vi "outPutOneTestCaseInCanFile.vi"(8 "error in":errorcluster, 10 "*varNoRepeatArr":string[](array[string]), 11 "secName":string) -> (0 "error out":errorcluster, 3 "oneTestCaseInCanFile":string[](array[string]))   [LabVIEW 2010]
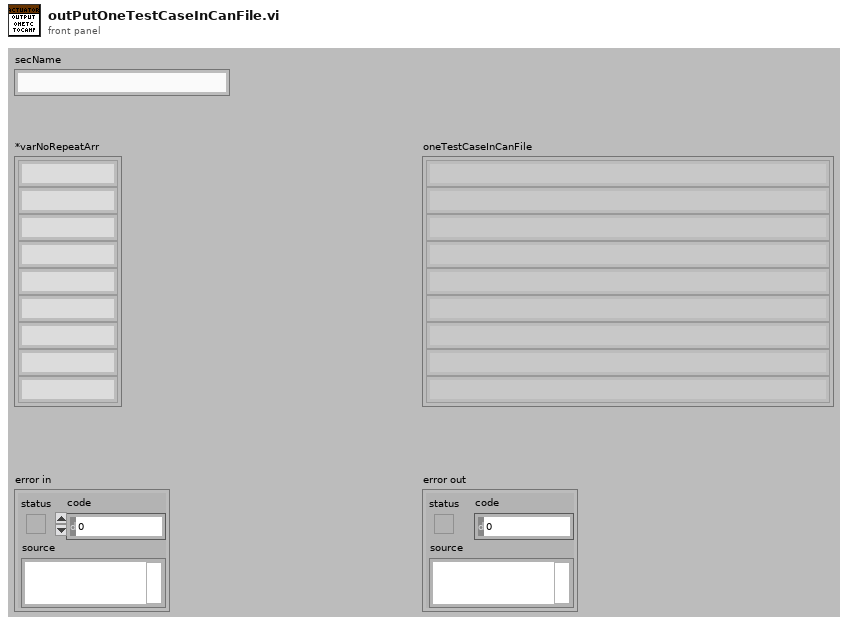
[diagram p1: front panel]
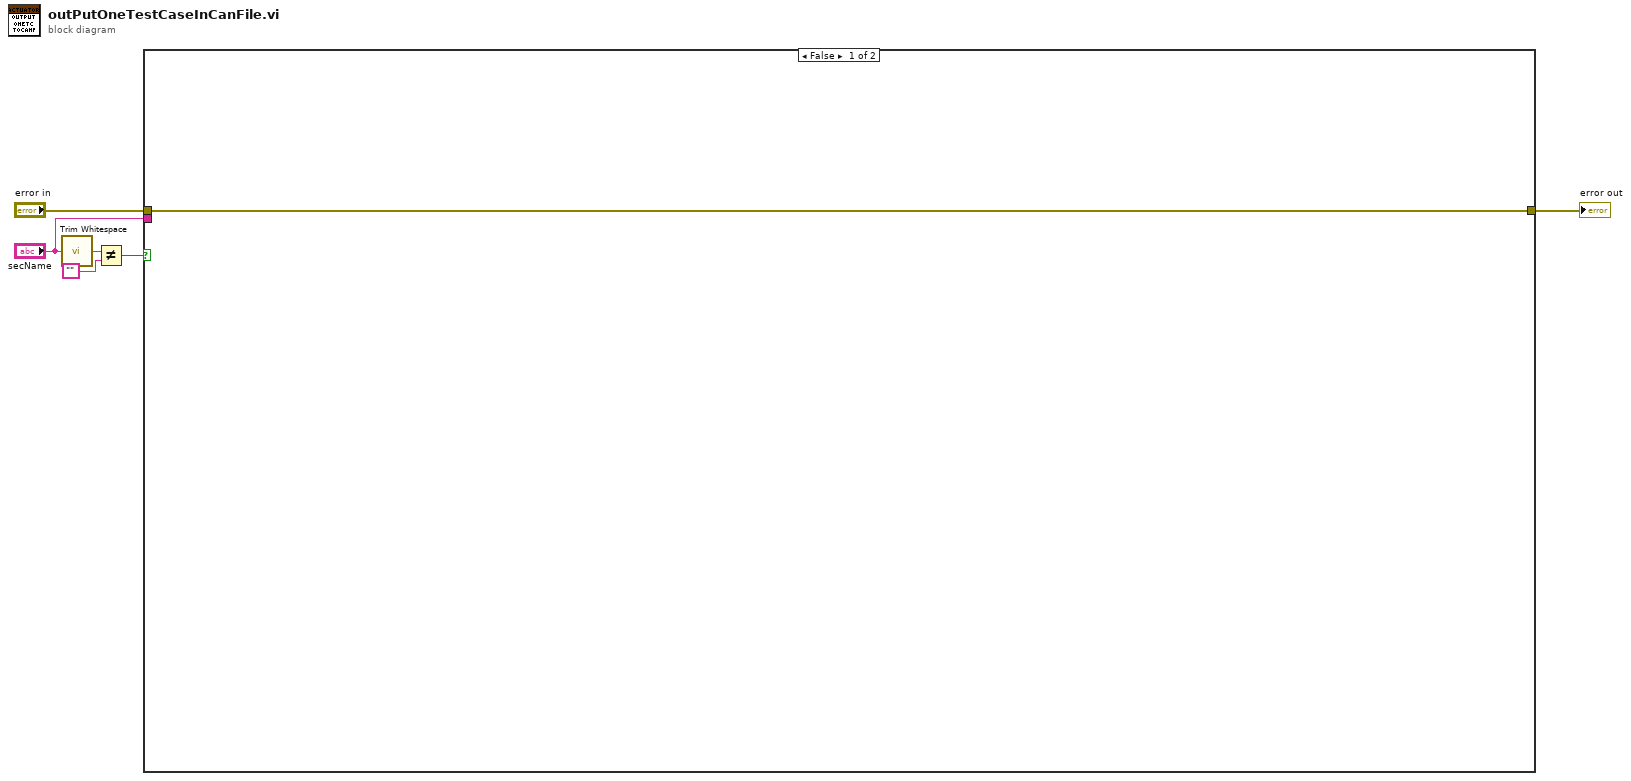
[diagram p0: block diagram]
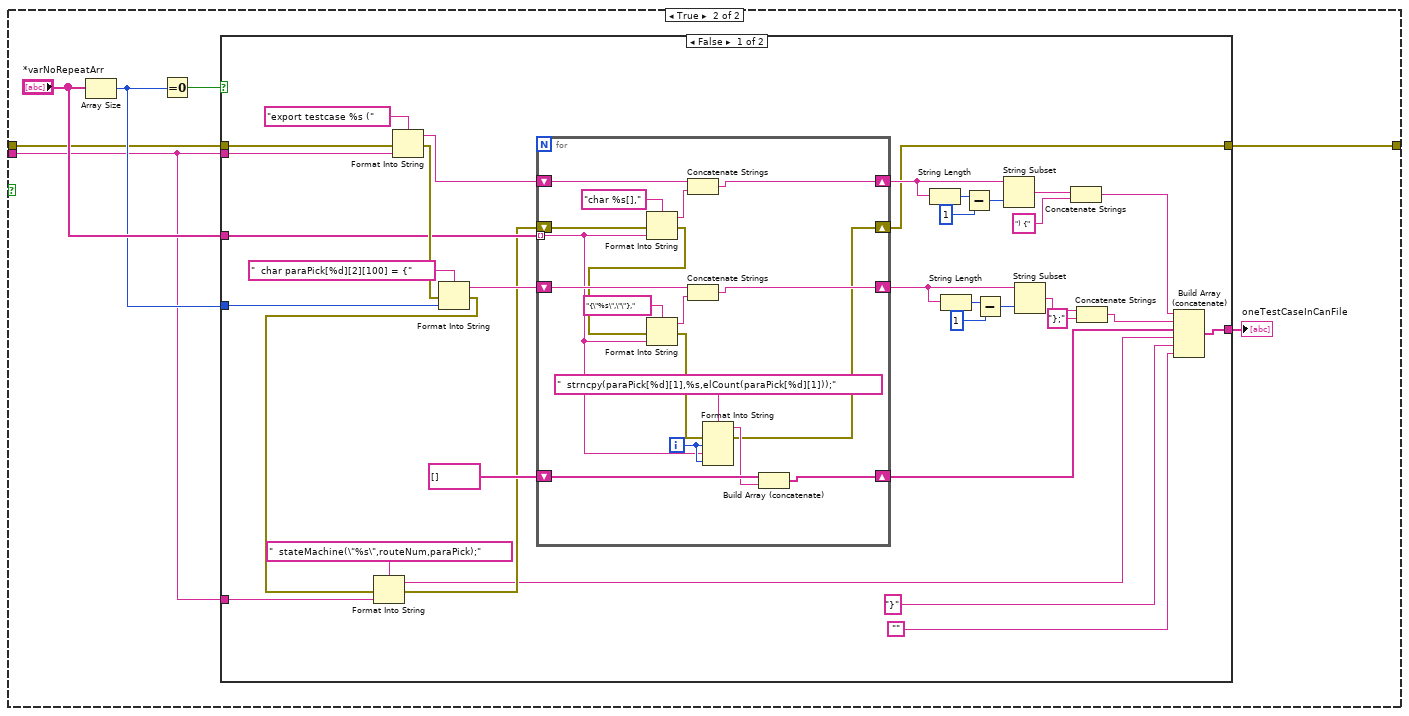
[diagram p2: hidden frame]
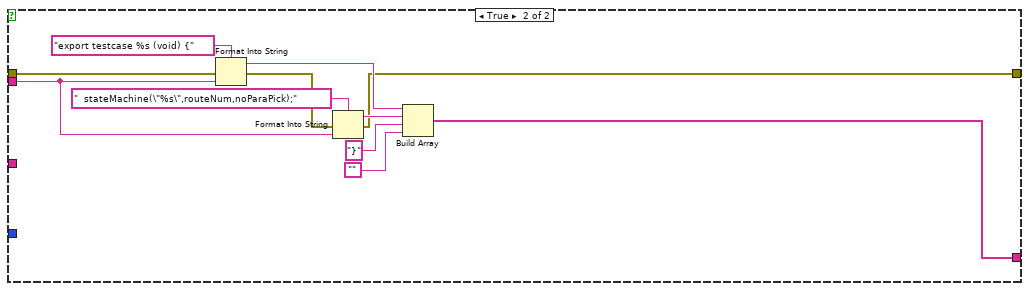
[diagram p3: hidden frame]
diagram:
  n1 = call <vilib>:"Trim Whitespace.vi"("string"="secName") -> ("trimmed string"=w6:string)  [unwired: 1 in]
  n2 = Not Equal?(x=w6, y="") -> (x != y?=w4:bool)
  n3 = case shown="False" w4 {
    tunnel: "secName" -> [_ w10]
    tunnel: "error in" -> [w7 w9]
    tunnel: [w7 w8] -> w1
    frame False {
    }
    frame True {
      n4 = Array Size(array="*varNoRepeatArr") -> (size(s)=w12:i32)
      n5 = Equal To 0?(x=w12) -> (x = 0?=w14:bool)
      n6 = case shown="False" w14 {
        tunnel: w10 -> [w47 w74]
        tunnel: w9 -> [w46 w73]
        tunnel: "*varNoRepeatArr" -> [w30 _]
        tunnel: w12 -> [w37 _]
        tunnel: w10 -> [w20 _]
        tunnel: [w19 w68] -> w11
        tunnel: [w18 w67] -> w8
        frame False {
          n7 = Format Into String(format string="export testcase %s (", error in=w46, w47) -> (resulting string=w45:string, error out=w39:errorcluster)  [unwired: 1 in]
          n8 = Format Into String(format string="  char paraPick[%d][2][100] = {", error in=w39, w37) -> (resulting string=w28:string, error out=w25:errorcluster)  [unwired: 1 in]
          n9 = Format Into String(format string="  stateMachine(\"%s\",routeNum,paraPick);", error in=w25, w20) -> (resulting string=w15:string, error out=w24:errorcluster)  [unwired: 1 in]
          n10 = for {
            tunnel: w30 -> [w56] mode=indexing
            shift-right: [w60] -> w29
            shift-left: w45 -> [w66]
            shift-right: [w65] -> w33
            shift-left: w28 -> [w59]
            shift-right: [w53] -> w21
            shift-left: string[] [] -> [w55]
            shift-right: [w49] -> w18
            shift-left: w24 -> [w52]
            i -> [w57]
            n11 = Format Into String(format string="char %s[],", error in=w52, w56) -> (resulting string=w61:string, error out=w51:errorcluster)  [unwired: 1 in]
            n12 = Format Into String(format string="{\"%s\",\"\"},", error in=w51, w56) -> (resulting string=w63:string, error out=w50:errorcluster)  [unwired: 1 in]
            n13 = Concatenate Strings(w66, w61) -> (w60:string)
            n14 = Concatenate Strings(w59, w63) -> (w65:string)
            n15 = Format Into String(format string="  strncpy(paraPick[%d][1],%s,elCount(paraPick[%d][1]));", error in=w50, w57, w56, w57) -> (resulting string=w54:string, error out=w49:errorcluster)  [unwired: 1 in]
            n16 = Build Array (concatenate)(w55, w54) -> (w53:string[])
          }
          n17 = String Length(string=w29) -> (length=w40:i32)
          n18 = String Length(string=w33) -> (length=w36:i32)
          n19 = Subtract(x=w40, y=1) -> (x-y=w42:i32)
          n20 = Subtract(x=w36, y=1) -> (x-y=w34:i32)
          n21 = String Subset(string=w29, length (rest)=w42) -> (substring=w43:string)  [unwired: 1 in]
          n22 = String Subset(string=w33, length (rest)=w34) -> (substring=w32:string)  [unwired: 1 in]
          n23 = Concatenate Strings(w43, ") {" ("sec")) -> (w23:string)
          n24 = Concatenate Strings(w32, "};" ("string")) -> (w22:string)
          n25 = Build Array (concatenate)(w23, w22, w21, w15, "}" ("string"), "") -> (w19:string[])
        }
        frame True {
          n26 = Format Into String(format string="export testcase %s (void) {", error in=w73, w74) -> (resulting string=w72:string, error out=w75:errorcluster)  [unwired: 1 in]
          n27 = Format Into String(format string="  stateMachine(\"%s\",routeNum,noParaPick);", error in=w75, w74) -> (resulting string=w71:string, error out=w67:errorcluster)  [unwired: 1 in]
          n28 = Build Array(w72, w71, "}", "") -> (w68:string[])
        }
      }
      "oneTestCaseInCanFile" <- w11
    }
  }
  "error out" <- w1
